vi "Parse_Valve.vi"(1 "Valve":string) -> (0 "Status":bool)   [LabVIEW 2016]
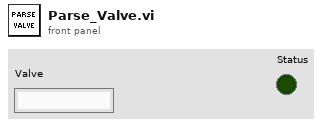
[diagram p1: front panel]
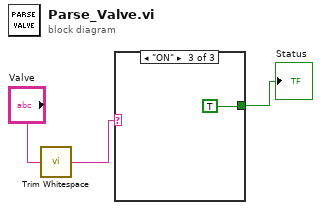
[diagram p0: block diagram]
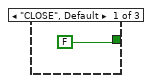
[diagram p2: hidden frame]
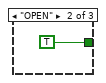
[diagram p3: hidden frame]
diagram:
  n1 = call <vilib>:"Trim Whitespace.vi"("string"="Valve") -> ("trimmed string"=w1:string)  [unwired: 1 in]
  n2 = case shown="\"ON\"" w1 {
    tunnel: [FALSE TRUE TRUE] -> w3
    frame "CLOSE", Default {
    }
    frame "OPEN" {
    }
    frame "ON" {
    }
  }
  "Status" <- w3
